vi "PID.vi"(6 "Derivative Time (Td)":sgl, 7 "Proportional Gain (Kc)":sgl, 9 "Process \nVariable":sgl, 10 "Setpoint":sgl, 11 "Integral Time (Ti)":sgl) -> (3 "Controller Output":sgl)   [LabVIEW 2013]
uses:
  <vilib>/rvi/Analysis/common/FxpNativeNode/niFpgaFxpNative.xnode
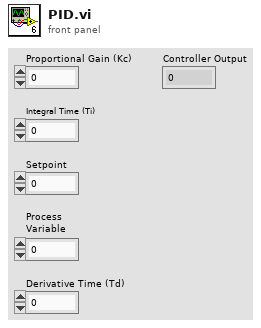
[diagram p1: front panel]
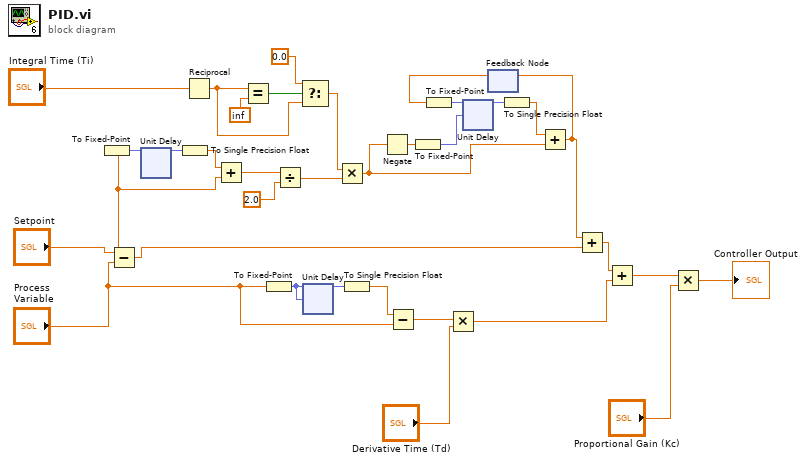
[diagram p0: block diagram]
diagram:
  n1 = Subtract(x="Setpoint", y="Process \nVariable") -> (x-y=w22:sgl)
  n2 = To Fixed-Point(number=w22) -> (fixed-point=w11:fxp<+/-,32,16>)  [unwired: 1 in]
  n3 = xnode ("Unit Delay")("input"=w11) -> ("output"=w12:fxp<+/-,32,16>)  [unwired: 2 in]
  n4 = To Single Precision Float(number=w12) -> (single precision float=w13:sgl)
  n5 = Reciprocal(x="Integral Time (Ti)") -> (1/x=w4:sgl)
  n6 = Add(x=w13, y=w22) -> (x+y=w9:sgl)
  n7 = Equal?(x=w4, y=sgl inf) -> (x = y?=w3:bool)
  n8 = To Fixed-Point(number="Process \nVariable") -> (fixed-point=w24:fxp<+/-,32,16>)  [unwired: 1 in]
  n9 = Divide(x=w9, y=sgl 2.0) -> (x/y=w7:sgl)
  n10 = Select(t=sgl 0.0, s=w3, f=w4) -> (s? t:f=w6:sgl)
  n11 = xnode ("Unit Delay")("initial condition"=w24, "input"=w24) -> ("output"=w23:fxp<+/-,32,16>)  [unwired: 1 in]
  n12 = Multiply(x=w6, y=w7) -> (x*y=w19:sgl)
  n13 = To Single Precision Float(number=w23) -> (single precision float=w25:sgl)
  n14 = Negate(x=w19) -> (-x=w17:sgl)
  n15 = Subtract(x=w25, y="Process \nVariable") -> (x-y=w27:sgl)
  n16 = To Fixed-Point(number=w17) -> (fixed-point=w16:fxp<+/-,32,16>)  [unwired: 1 in]
  n17 = Multiply(x=w27, y="Derivative Time (Td)") -> (x*y=w30:sgl)
  n18 = feedback #1() -> (w20:sgl)  [unwired: 1 in]
  n19 = To Fixed-Point(number=w20) -> (fixed-point=w14:fxp<+/-,32,16>)  [unwired: 1 in]
  n20 = xnode ("Unit Delay")("initial condition"=w16, "input"=w14) -> ("output"=w15:fxp<+/-,32,16>)  [unwired: 1 in]
  n21 = To Single Precision Float(number=w15) -> (single precision float=w18:sgl)
  n22 = Add(x=w18, y=w19) -> (x+y=w21:sgl)
  n23 = feedback-in #1(w21) -> ()
  n24 = Add(x=w21, y=w22) -> (x+y=w29:sgl)
  n25 = Add(x=w29, y=w30) -> (x+y=w32:sgl)
  n26 = Multiply(x=w32, y="Proportional Gain (Kc)") -> (x*y=→"Controller Output":sgl)
